vi "Initialize Hardware References.vi"(8 "error in (no error)":errorcluster, 11 "Hardware Resources in":T1={"AI"={"task name"="", "task_ref"="", "physical channels"="Dev1/ai0:7", "channels config"={"input terminal configuration"=0, "minimum value"=-5.0, "maximum value"=5.0}, "rate"=1000.0}, "conversions"={"ai0"={"a"=0.0, "b"=0.0}, "ai1"={"a"=0.0, "b"=0.0}, "ai2"={"a"=0.0, "b"=0.0}, "ai3"={"a"=0.0, "b"=0.0}, "ai4"={"a"=0.0, "b"=0.0}}, "compteur 0"={"task name"="CTR", "task_ref"="", "ctr"="Dev1/ctr0:3", "coeff"=4000.0}, "compteur 1"={"task name"="CTR1", "task_ref"="", "ctr"="Dev1/ctr1", "coeff"=4000.0}, "compteur 2"={"task name"="CTR2", "task_ref"="", "ctr"="Dev1/ctr2", "coeff"=4000.0}, "compteur 3"={"task name"="CTR3", "task_ref"="", "ctr"="Dev1/ctr3", "coeff"=4000.0}} {"compteur 3"."coeff" format="%0.2f"; "compteur 2"."coeff" format="%0.2f"; "compteur 1"."coeff" format="%0.2f"; "compteur 0"."coeff" format="%0.2f"; "AI"."rate" format="%0.2f"; "AI"."channels config"."input terminal configuration" items=["Default"=-1, "RSE"=10083, "NRSE"=10078, "Differential"=10106, "Pseudodifferential"=12529]}) -> (0 "error out":errorcluster, 3 "Hardware Resources out":T1={"AI"={"task name"="", "task_ref"="", "physical channels"="Dev1/ai0:7", "channels config"={"input terminal configuration"=0, "minimum value"=-5.0, "maximum value"=5.0}, "rate"=1000.0}, "conversions"={"ai0"={"a"=0.0, "b"=0.0}, "ai1"={"a"=0.0, "b"=0.0}, "ai2"={"a"=0.0, "b"=0.0}, "ai3"={"a"=0.0, "b"=0.0}, "ai4"={"a"=0.0, "b"=0.0}}, "compteur 0"={"task name"="CTR", "task_ref"="", "ctr"="Dev1/ctr0:3", "coeff"=4000.0}, "compteur 1"={"task name"="CTR1", "task_ref"="", "ctr"="Dev1/ctr1", "coeff"=4000.0}, "compteur 2"={"task name"="CTR2", "task_ref"="", "ctr"="Dev1/ctr2", "coeff"=4000.0}, "compteur 3"={"task name"="CTR3", "task_ref"="", "ctr"="Dev1/ctr3", "coeff"=4000.0}} {"compteur 3"."coeff" format="%0.2f"; "compteur 2"."coeff" format="%0.2f"; "compteur 1"."coeff" format="%0.2f"; "compteur 0"."coeff" format="%0.2f"; "AI"."rate" format="%0.2f"; "AI"."channels config"."input terminal configuration" items=["Default"=-1, "RSE"=10083, "NRSE"=10078, "Differential"=10106, "Pseudodifferential"=12529]})   [LabVIEW 2014, in "PLS Acquisition.lvlib"]
doc: "Initialize the hardware references."
uses:
  PLS Acquisition.lvlib
  Hardware Configuration.ctl
  Settings/conversion.ctl
  <vilib>/DAQmx/create/channels.llb/DAQmx Create Channel (CI-Count Edges).vi
  <vilib>/DAQmx/create/channels.llb/DAQmx Create Channel (AI-Voltage-Basic).vi
  <vilib>/DAQmx/configure/timing.llb/DAQmx Timing (Sample Clock).vi
  <resource>/objmgr/daqmx.rc
  Settings/PLS Settings.lvlib
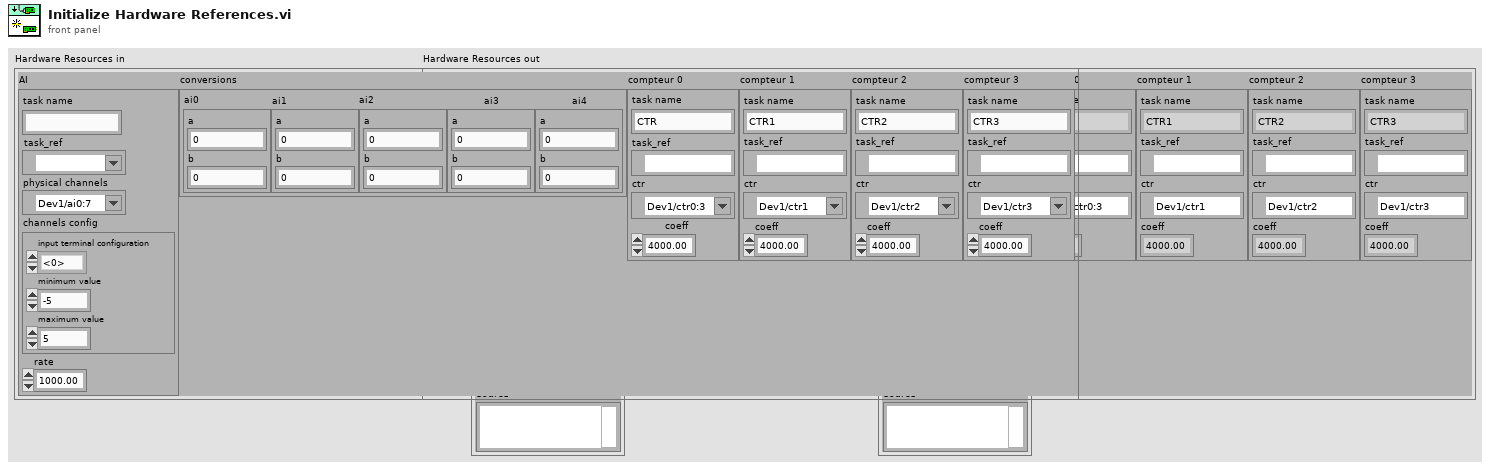
[diagram p1: front panel]
types:
  T1 = typedef "PLS Acquisition.lvlib/Hardware Configuration.ctl" = cluster{"AI":cluster{"task name":string, "task_ref":refnum<k21>, "physical channels":tag, "channels config":cluster{"input terminal configuration":i32, "minimum value":dbl, "maximum value":dbl}, "rate":dbl}, "conversions":cluster{"ai0":T2, "ai1":T2, "ai2":T2, "ai3":T2, "ai4":T2}, "compteur 0":cluster{"task name":string, "task_ref":refnum<k21>, "ctr":tag, "coeff":dbl}, "compteur 1":cluster{"task name":string, "task_ref":refnum<k21>, "ctr":tag, "coeff":dbl}, "compteur 2":cluster{"task name":string, "task_ref":refnum<k21>, "ctr":tag, "coeff":dbl}, "compteur 3":cluster{"task name":string, "task_ref":refnum<k21>, "ctr":tag, "coeff":dbl}}
  T2 = typedef "PLS Settings.lvlib/conversion.ctl" = cluster{"a":dbl, "b":dbl}
  T3 = cluster{"task name":string, "task_ref":refnum<k21>, "physical channels":tag, "channels config":cluster{"input terminal configuration":i32, "minimum value":dbl, "maximum value":dbl}, "rate":dbl}
  T4 = cluster{"task name":string, "task_ref":refnum<k21>, "ctr":tag, "coeff":dbl}
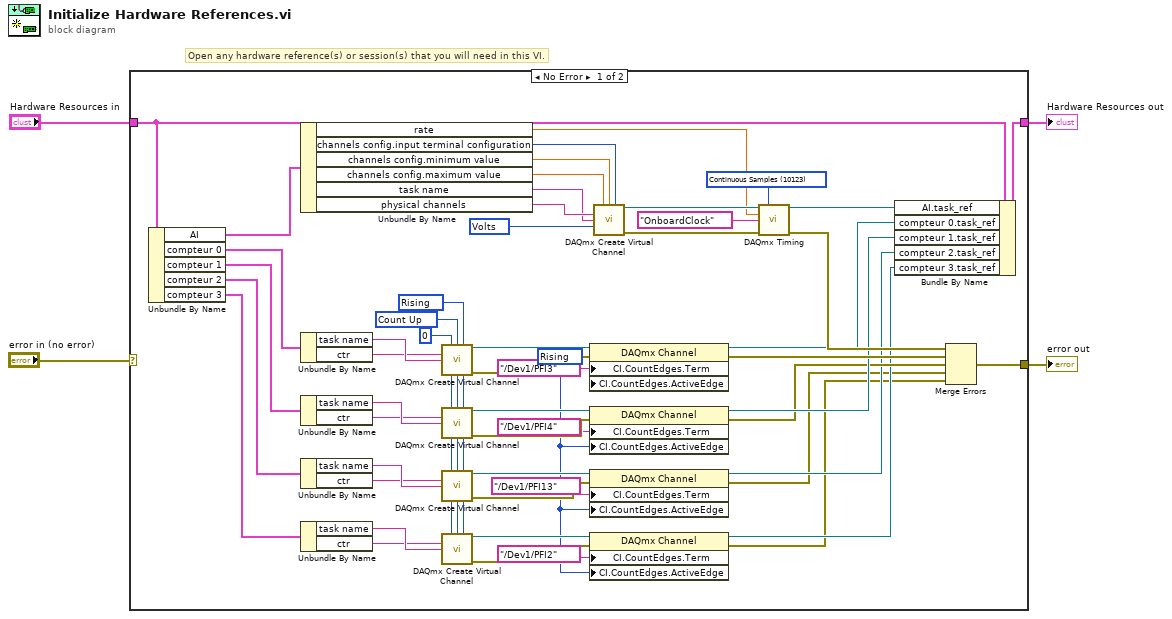
[diagram p0: block diagram]
diagram:
  # "Open any hardware reference(s) or session(s) that you will need in this VI."
  n1 = case shown="No Error" "error in (no error)" {
    selector: "error in (no error)" -> [_ w58]
    tunnel: [w42 w58] -> w3
    tunnel: "Hardware Resources in" -> [w45 w59]
    tunnel: [w44 w59] -> w1
    frame No Error {
      w5 = 10280 items=["Rising"=10280, "Falling"=10171] ("CI.CountEdges.ActiveEdge")
      w40 = 10280 items=["Rising"=10280, "Falling"=10171] ("edge")
      w39 = 10128 items=["Count Up"=10128, "Count Down"=10124, "Externally Controlled"=10326] ("count direction")
      w38 = u32 0 ("initial count")
      w49 = 10123 items=["Finite Samples"=10178, "Continuous Samples"=10123, "Hardware Timed Single Point"=12522] ("sample mode")
      w57 = 10348 items=["Volts"=10348, "From Custom Scale"=10065] ("units")
      n2 = Unbundle By Name(w45) -> ("AI"=w46:T3, "compteur 0"=w37:T4, "compteur 1"=w34:T4, "compteur 2"=w33:T4, "compteur 3"=w32:T4)
      n3 = Unbundle By Name(w46) -> ("rate"=w48:dbl, "channels config.input terminal configuration"=w54:i32, "channels config.minimum value"=w55:dbl, "channels config.maximum value"=w56:dbl, "task name"=w50:string, "physical channels"=w51:tag)
      n4 = Unbundle By Name(w37) -> ("task name"=w36:string, "ctr"=w35:tag)
      n5 = Unbundle By Name(w34) -> ("task name"=w31:string, "ctr"=w28:tag)
      n6 = Unbundle By Name(w33) -> ("task name"=w30:string, "ctr"=w27:tag)
      n7 = Unbundle By Name(w32) -> ("task name"=w29:string, "ctr"=w26:tag)
      n8 = call-poly <vilib>:"DAQmx Create Virtual Channel.vi"("initial count"=w38, "count direction"=w39, "edge"=w40, "counter"=w35, "name to assign"=w36) -> ("task out"=w25:refnum<k21>, "error out"=w23:errorcluster)  [unwired: 9 in]
      n9 = call-poly <vilib>:"DAQmx Create Virtual Channel.vi"("initial count"=w38, "count direction"=w39, "edge"=w40, "counter"=w28, "name to assign"=w31) -> ("task out"=w20:refnum<k21>, "error out"=w18:errorcluster)  [unwired: 9 in]
      n10 = call-poly <vilib>:"DAQmx Create Virtual Channel.vi"("initial count"=w38, "count direction"=w39, "edge"=w40, "counter"=w27, "name to assign"=w30) -> ("task out"=w16:refnum<k21>, "error out"=w10:errorcluster)  [unwired: 9 in]
      n11 = call-poly <vilib>:"DAQmx Create Virtual Channel.vi"("initial count"=w38, "count direction"=w39, "edge"=w40, "counter"=w26, "name to assign"=w29) -> ("task out"=w14:refnum<k21>, "error out"=w12:errorcluster)  [unwired: 9 in]
      n12 = property class="DAQmx Channel"(reference=w25, error in=w23, "CI.CountEdges.Term"=tag "/Dev1/PFI3", "CI.CountEdges.ActiveEdge"=w5) -> (reference out=w24:refnum<k21>, error out=w22:errorcluster)
      n13 = property class="DAQmx Channel"(reference=w20, error in=w18, "CI.CountEdges.Term"=tag "/Dev1/PFI4", "CI.CountEdges.ActiveEdge"=w5) -> (reference out=w19:refnum<k21>, error out=w17:errorcluster)
      n14 = property class="DAQmx Channel"(reference=w16, error in=w10, "CI.CountEdges.Term"=tag "/Dev1/PFI13", "CI.CountEdges.ActiveEdge"=w5) -> (reference out=w15:refnum<k21>, error out=w9:errorcluster)
      n15 = property class="DAQmx Channel"(reference=w14, error in=w12, "CI.CountEdges.Term"=tag "/Dev1/PFI2", "CI.CountEdges.ActiveEdge"=w5) -> (reference out=w13:refnum<k21>, error out=w11:errorcluster)
      n16 = call-poly <vilib>:"DAQmx Create Virtual Channel.vi"("maximum value"=w56, "minimum value"=w55, "input terminal configuration"=w54, "physical channels"=w51, "name to assign"=w50, "units"=w57) -> ("task out"=w53:refnum<k21>, "error out"=w52:errorcluster)  [unwired: 8 in]
      n17 = call-poly <vilib>:"DAQmx Timing.vi"("task/channels in"=w53, "sample mode"=w49, "rate"=w48, "source"=tag "OnboardClock", "error in"=w52) -> ("task out"=w43:refnum<k21>, "error out"=w41:errorcluster)  [unwired: 9 in]
      n18 = Bundle By Name(cluster=w45, "AI.task_ref"=w43, "compteur 0.task_ref"=w24, "compteur 1.task_ref"=w19, "compteur 2.task_ref"=w15, "compteur 3.task_ref"=w13) -> (w44:T1)
      n19 = Merge Errors(w41, w22, w17, w9, w11) -> (w42:errorcluster)
    }
    frame Error {
    }
  }
  "Hardware Resources out" <- w1
  "error out" <- w3
